vi "Using Temperature.vi"() -> ()   [LabVIEW 2015]
panel:
  in  "Stop Button":bool
  out "Chart":dbl(graph)
  in  "Delay Multiplier":dbl(knob) min=0.0 max=2.0 step=0.1 scale=0.0..2.0
  in  "Numeric":i32
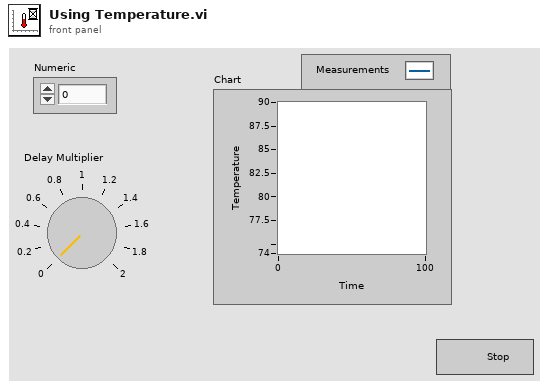
[diagram p1: front panel]
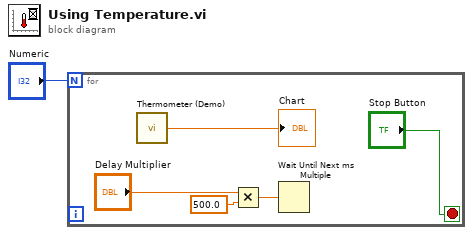
[diagram p0: block diagram]
diagram:
  n1 = for {
    N: "Numeric" -> [_]
    stop <- "Stop Button" stop-if-true
    n2 = call "Thermometer (Demo).vi"() -> ("Temperature Value"=→"Chart":dbl)  [unwired: 1 in]
    n3 = Multiply(x="Delay Multiplier", y=500.0) -> (x*y=w4:dbl)
    n4 = Wait Until Next ms Multiple(millisecond multiple=w4) -> ()  [unwired: 1 out]
  }
